vi "Creator Attributes.vi"(11 "Base Actor in":refnum<class "Base Actor.lvclass">) -> (2 "Creator Attributes":T1)   [LabVIEW 2020, in "jettl.lvlib" / "Actor.lvlib" / "Base Actor.lvclass"]
uses:
  Base Actor.lvclass
  Attributes.ctl
  Msg/Msg.lvclass
  Implemented Msgs.ctl
  Base Actor.lvclass/Base Actor.ctl
  Actor.lvlib
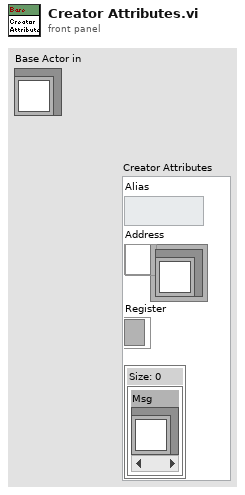
[diagram p1: front panel]
types:
  T1 = typedef "jettl.lvlib/Actor.lvlib/Attributes.ctl" = cluster{"Alias":string, "Address":refnum<user-event>, "Register":refnum<event-registration>, "Implemented Msgs":T2}
  T2 = typedef "jettl.lvlib/Actor.lvlib/Implemented Msgs.ctl" = set{refnum<class "Msg.lvclass">}
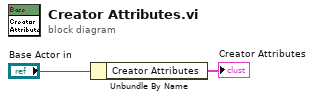
[diagram p0: block diagram]
diagram:
  n1 = Unbundle By Name("Base Actor in") -> ("Creator Attributes"=→"Creator Attributes":T1)
